vi "Message Callback.vi"(7 "Owner":refnum<class>, 11 "Message":refnum<class "Message.lvclass">) -> (0 "error out":errorcluster)   [LabVIEW 2020, in "LV Server.lvclass"]
uses:
  LV Server.lvclass
  lv-msg-simple/Stream-Simple-Msg/Message/Message.lvclass
  Common/Message ID.ctl
  Common/Common.lvlib
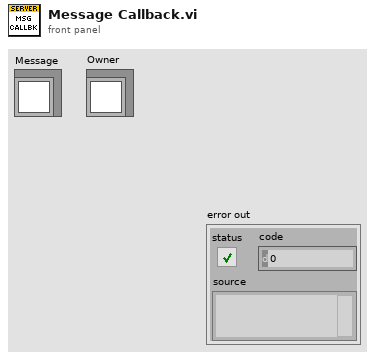
[diagram p1: front panel]
types:
  T1 = typedef "Common.lvlib/Message ID.ctl" = enum16{"Timer State", "Timer Value", "Timer Start", "Timer Pause", "Timer Reset", "Timer Init"}
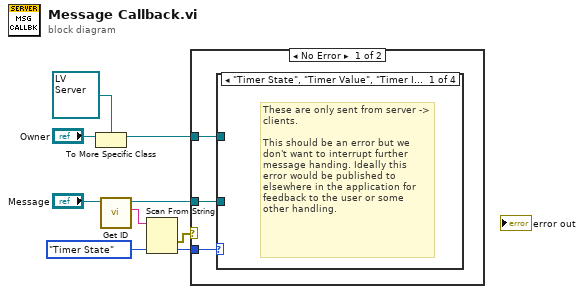
[diagram p0: block diagram]
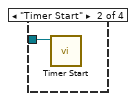
[diagram p2: hidden frame]
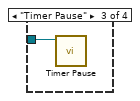
[diagram p3: hidden frame]
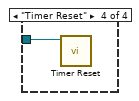
[diagram p4: hidden frame]
diagram:
  n1 = To More Specific Class(target class=refnum<class "LV Server.lvclass"> refnum ("LV Server.lvclass"), reference="Owner") -> (specific class reference=w1:refnum<class "LV Server.lvclass">)  [unwired: 1 in, 1 out]
  n2 = call "Get ID.vi"("Message in"="Message") -> ("ID"=w6:string, "Message out"=w2:refnum<class "Message.lvclass">)  [unwired: 8 in, 1 out]
  n3 = Scan From String(input string=w6, default 1=Message_ID."Timer State" ("Message ID")) -> (error out=w4:errorcluster, output 1=w3:T1)  [unwired: 3 in, 2 out]
  n4 = case shown="No Error" w4 {
    tunnel: w3 -> [w10 _]
    tunnel: w2 -> [w12 _]
    tunnel: w1 -> [w11 _]
    frame No Error {
      n5 = case shown="\"Timer State\", \"Timer Value\", \"Timer Init\"" w10 {
        tunnel: w12 -> [_ _ _ _]
        tunnel: w11 -> [_ w13 w14 w15]
        frame "Timer State", "Timer Value", "Timer Init" {
          # "These are only sent from server -> clients.\n\nThis should be an error but we don't want to interrupt further message handing. Ideally this error would be published to elsewhere in the application for feedback to the user or some other handling."
        }
        frame "Timer Start" {
          n6 = call "Timer Start.vi"("LV Server in"=w13) -> ()  [unwired: 9 in, 2 out]
        }
        frame "Timer Pause" {
          n7 = call "Timer Pause.vi"("LV Server in"=w14) -> ()  [unwired: 9 in, 2 out]
        }
        frame "Timer Reset" {
          n8 = call "Timer Reset.vi"("LV Server in"=w15) -> ()  [unwired: 9 in, 2 out]
        }
      }
    }
    frame Error {
    }
  }
